vi "Get Boolean.vi"(8 "error in (no error)":errorcluster, 11 "Test Process In":refnum<class "Test Process.lvclass">) -> (0 "error out":errorcluster, 2 "Boolean":bool, 3 "Test Process Out":refnum<class "Test Process.lvclass">)   [LabVIEW 2020, in "Test Process.lvclass"]
uses:
  Test Process.lvclass
  Test Process.lvclass/Test Process.ctl
  <vilib>/Astemes/Triarc Framework/Process/Process.lvclass
  C:/Program Files (x86)/National Instruments/LabVIEW 2020/vi.lib/Astemes/Triarc Framework/Process/Process.lvclass
  C:/Program Files (x86)/National Instruments/LabVIEW 2020/vi.lib/Astemes/Triarc Framework/Base/Base.lvclass
  C:/Program Files (x86)/National Instruments/LabVIEW 2020/vi.lib/Astemes/Triarc Framework/Error Handler Interface/Error Handler Interface.lvclass
  C:/Program Files (x86)/National Instruments/LabVIEW 2020/vi.lib/Astemes/Triarc Framework/Logging/Logging.lvclass
  C:/Users/anton/Documents/GitHub/triarc-debugger/test/Test Process/Test Process.lvclass
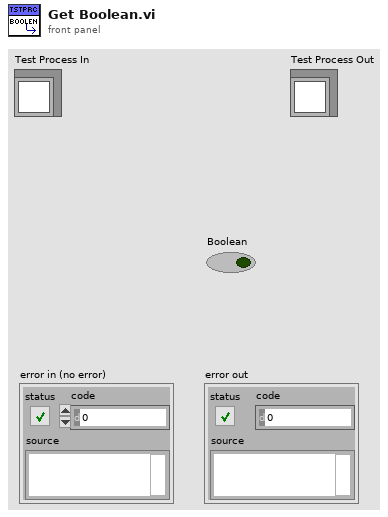
[diagram p1: front panel]
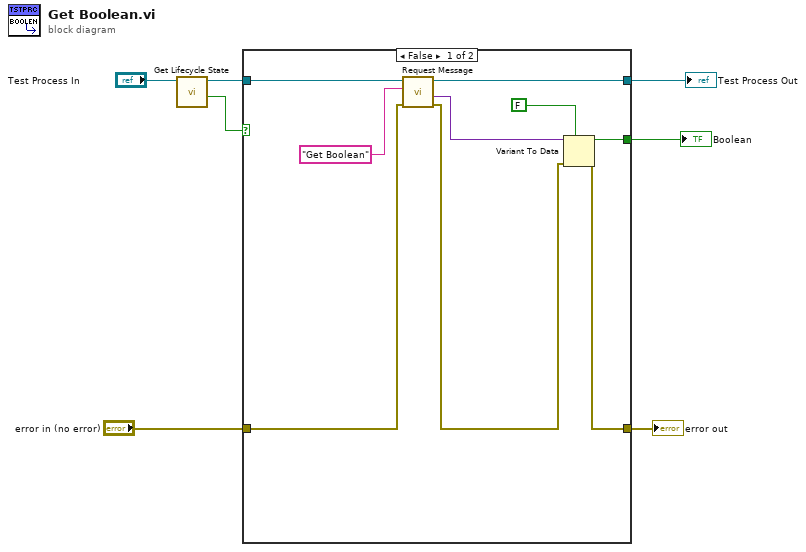
[diagram p0: block diagram]
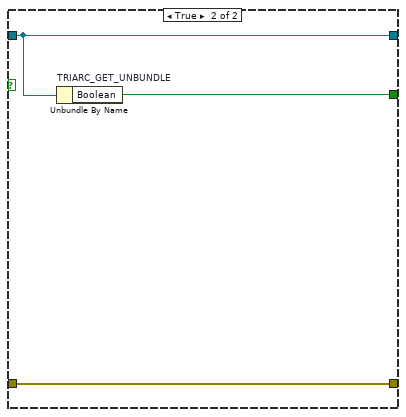
[diagram p2: hidden frame]
diagram:
  n1 = call <vilib>:"Get Lifecycle State.vi"("Process In"="Test Process In") -> ("In Process Loop?"=w2:bool, "Process Out"=w6:refnum<class "Test Process.lvclass">)  [unwired: 7 in, 2 out]
  n2 = case shown="False" w2 {
    tunnel: w6 -> [w16 w19]
    tunnel: [w15 w19] -> w5
    tunnel: "error in (no error)" -> [w14 w18]
    tunnel: [w11 w18] -> w4
    tunnel: [w9 w17] -> w3
    frame False {
      n3 = call <vilib>:"Request Message.vi"("error in (no error)"=w14, "Request Message"="Get Boolean" ("API Message"), "Process In"=w16) -> ("error out"=w12:errorcluster, "Response Message Data"=w13:variant, "Process Out"=w15:refnum<class "Test Process.lvclass">)  [unwired: 4 in, 2 out]
      n4 = Variant To Data(error in=w12, type=FALSE ("Type Speifier"), Variant=w13) -> (data=w9:bool, error out=w11:errorcluster)
    }
    frame True {
      n5 = Unbundle By Name "TRIARC_GET_UNBUNDLE"(w19) -> ("Boolean"=w17:bool)
    }
  }
  "error out" <- w4
  "Test Process Out" <- w5
  "Boolean" <- w3
